vi "coding(4800).vi"(7 "Кадр на вход\nкодера":bool[](array[boolean])) -> (8 "Поток кодированных \nбитов":bool[](array[boolean]))   [LabVIEW 2013]
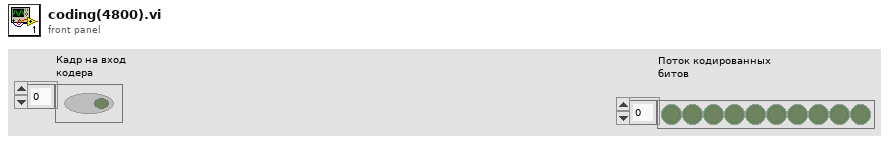
[diagram p1: front panel]
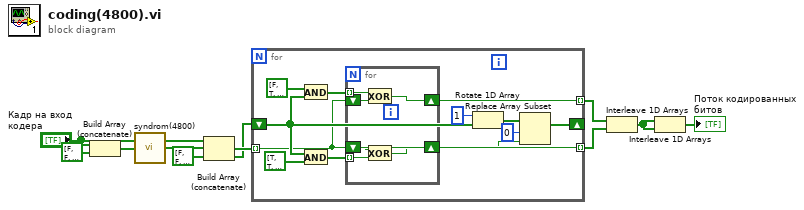
[diagram p0: block diagram]
diagram:
  w6 = bool[] [FALSE, FALSE, FALSE, FALSE, FALSE, FALSE, FALSE, FALSE] ("array")
  n1 = Build Array (concatenate)("Кадр на вход\nкодера", bool[] [FALSE, FALSE, FALSE, FALSE, FALSE, FALSE, FALSE, FALSE] ("array")) -> (w8:bool[])
  n2 = call "syndrom(4800).vi"("Кадр для  вычисления \nсиндрома"=w8) -> ("Синдром"=w9:bool[])  [unwired: 14 in]
  n3 = Build Array (concatenate)("Кадр на вход\nкодера", w9, w6) -> (w10:bool[])
  n4 = for {
    tunnel: w10 -> [w11] mode=indexing
    shift-right: [w13] -> _
    shift-left: w6 -> [w12]
    tunnel: [w18] -> w4 mode=indexing
    tunnel: [w17] -> w3 mode=indexing
    n5 = And(x=bool[] [FALSE, TRUE, TRUE, TRUE, FALSE, FALSE, FALSE, TRUE], y=w12) -> (x .and. y?=w20:bool[])
    n6 = And(x=w12, y=bool[] [TRUE, TRUE, TRUE, FALSE, TRUE, FALSE, TRUE, TRUE]) -> (x .and. y?=w19:bool[])
    n7 = for {
      tunnel: w20 -> [w28] mode=indexing
      tunnel: w19 -> [w27] mode=indexing
      shift-right: [w26] -> w18
      shift-left: w11 -> [w25]
      shift-right: [w24] -> w17
      shift-left: w11 -> [w23]
      n8 = Exclusive Or(1:w25, 2:w28) -> (0:w26:bool)
      n9 = Exclusive Or(1:w27, 2:w23) -> (0:w24:bool)
    }
    n10 = Rotate 1D Array(1:w12, 2:1 ("n")) -> (0:w15:bool[])
    n11 = Replace Array Subset(array=w15, new element=w11, index=0) -> (w13:bool[])
  }
  n12 = Interleave 1D Arrays(w4, w3) -> (w2:bool[])
  n13 = Interleave 1D Arrays(w2, w2) -> (→"Поток кодированных \nбитов":bool[])
